vi "Write free space.vi"(8 "error in (no error)":errorcluster, 10 "free space":u32, 11 "tCRD Data in":refnum<class "tCRD Data.lvclass">) -> (0 "error out":errorcluster, 3 "tCRD Data out":refnum<class "tCRD Data.lvclass">)   [LabVIEW 2015, in "tCRD Data.lvclass"]
uses:
  tCRD Data.lvclass
  tCRD Data.lvclass/tCRD Data.ctl
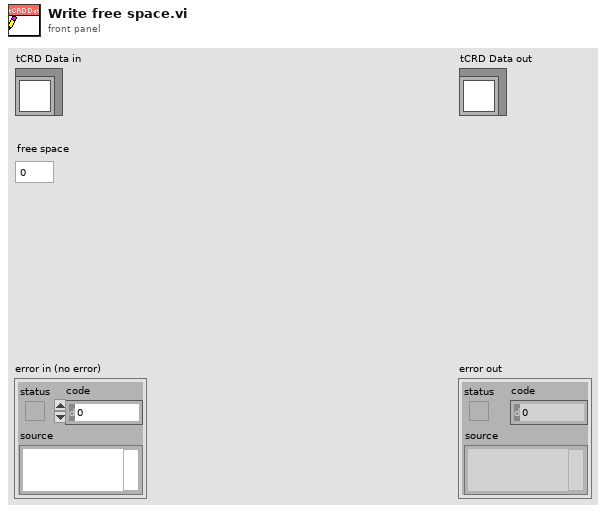
[diagram p1: front panel]
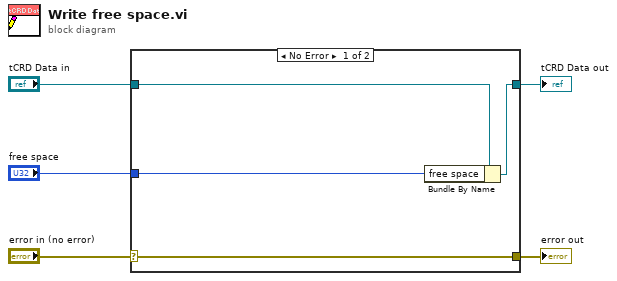
[diagram p0: block diagram]
diagram:
  n1 = case shown="No Error" "error in (no error)" {
    selector: "error in (no error)" -> [w9 w10]
    tunnel: [w9 w10] -> w4
    tunnel: [w7 w11] -> w2
    tunnel: "tCRD Data in" -> [w8 w11]
    tunnel: "free space" -> [w6 _]
    frame No Error {
      n2 = Bundle By Name(cluster=w8, "free space"=w6) -> (w7:refnum<class "tCRD Data.lvclass">)
    }
    frame Error {
    }
  }
  "error out" <- w4
  "tCRD Data out" <- w2
